vi "test.vi"() -> ()   [LabVIEW 2022 SP3]
uses:
  <vilib>/Instr/_visa.llb/VISA Configure Serial Port (Instr).vi
panel:
  out "连接的字符串":string
  in  "baud rate (9600)":u32=9600 caption="波特率(9600)"
  in  "VISA resource name":refnum<visa-resource-name> caption="VISA资源名称"
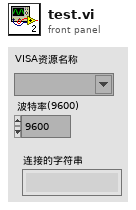
[diagram p1: front panel]
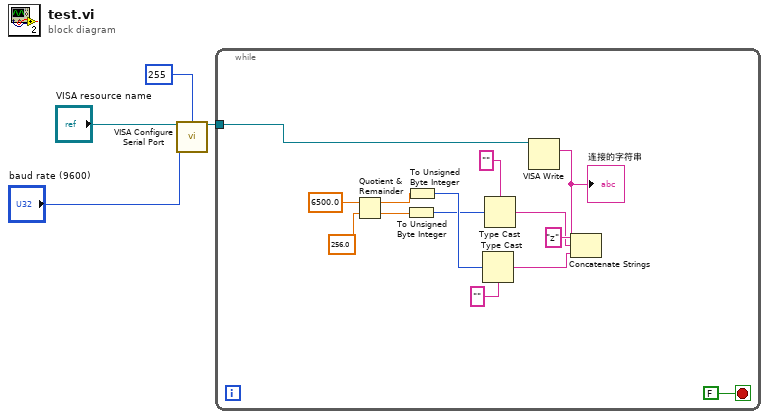
[diagram p0: block diagram]
diagram:
  n1 = call-poly "VISA Configure Serial Port"("VISA resource name"="VISA resource name", "termination char\n(0xA = '\\n' = LF)"=u16 255 ("termination char\n(0xA = '\\n' = LF)"), "baud rate (9600)"="baud rate (9600)") -> ("VISA resource name out"=w1:refnum<visa-resource-name>)  [unwired: 11 in, 1 out]
  n2 = while {
    tunnel: w1 -> [w18]
    stop <- FALSE stop-if-true
    n3 = Quotient & Remainder(x=6500.0, y=256.0) -> (x-y*floor(x/y)=w14:dbl, floor(x/y)=w15:dbl)
    n4 = To Unsigned Byte Integer(number=w15) -> (unsigned 8bit integer=w10:u8)
    n5 = To Unsigned Byte Integer(number=w14) -> (unsigned 8bit integer=w13:u8)
    n6 = Type Cast(type="" ("类型"), x=w13) -> (*(type *) &x=w7:string)
    n7 = Type Cast(type="" ("类型"), x=w10) -> (*(type *) &x=w8:string)
    n8 = Concatenate Strings("z" ("字符串"), w8, w7) -> (w6:string)
    "连接的字符串" <- w6
    n9 = VISA Write(VISA resource name=w18, write buffer=w6) -> ()  [unwired: 1 in, 3 out]
  }
